vi "Get Error.vi"(8 "error in":errorcluster, 11 "LogRecord in":refnum<class "LogRecord.lvclass">) -> (0 "error out":errorcluster, 2 "Error":errorcluster, 3 "LogRecord out":refnum<class "LogRecord.lvclass">)   [LabVIEW 2016, in "hse-logger.lvlib" / "LogRecord.lvclass"]
doc: "Returns the error-cluster from the LogRecord.\n\n____\n(c) HAMPEL SOFTWARE ENGINEERING"
uses:
  LogRecord.lvclass
  LogRecord.lvclass/LogRecord.ctl
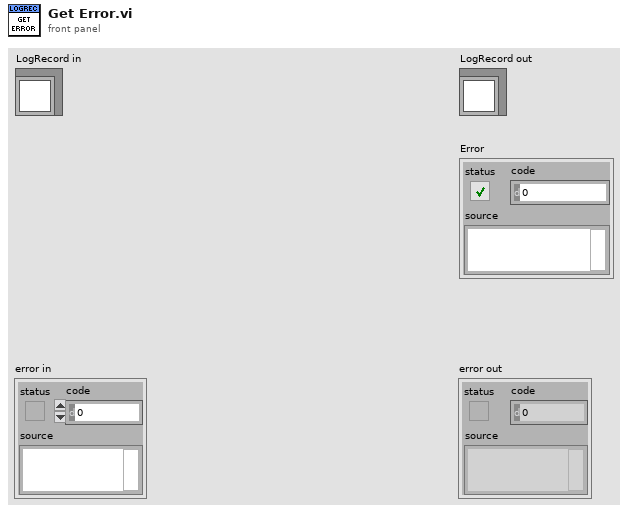
[diagram p1: front panel]
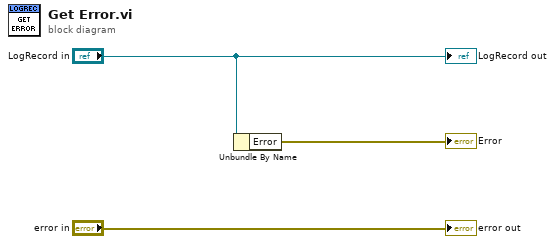
[diagram p0: block diagram]
diagram:
  n1 = Unbundle By Name("LogRecord in") -> ("Error"=→"Error":errorcluster)
  "error out" <- "error in"
  "LogRecord out" <- "LogRecord in"
